vi "MasterAcquisitionFile_PCO_IOS_MultiWavelength.vi"() -> ()   [LabVIEW 2020]
uses:
  <userlib>/PCO LabVIEW 5.0.0/pco.camera/Controls/binning.ctl
  <vilib>/vision/driver/IMAQdx.llb/IMAQdx Acquisition Mode.ctl
  <vilib>/vision/driver/IMAQdx.llb/IMAQdx Camera Control Mode.ctl
  <vilib>/userDefined/High Color/IMAQdx.ctl
  <userlib>/PCO LabVIEW 5.0.0/pco.camera/Camera.lvclass
  <vilib>/vision/driver/IMAQdx.llb/IMAQdx Buffer Number Mode.ctl
  <vilib>/DAQmx/write.llb/DAQmx Write (Digital 1D Wfm NChan NSamp).vi
  <vilib>/DAQmx/write.llb/DAQmx Write (Digital Bool 1Line 1Point).vi
  <vilib>/DAQmx/read.llb/DAQmx Read (Analog 1D Wfm NChan NSamp).vi
  <vilib>/Waveform/DWDTOps.llb/DWDT Digital to Boolean Array.vi
  <vilib>/DAQmx/create/channels.llb/DAQmx Create Channel (CO-Pulse Generation-Frequency).vi
  <vilib>/DAQmx/configure/timing.llb/DAQmx Timing (Implicit).vi
  <vilib>/DAQmx/create/channels.llb/DAQmx Create Channel (AI-Voltage-Basic).vi
  <vilib>/DAQmx/configure/timing.llb/DAQmx Timing (Sample Clock).vi
  <vilib>/DAQmx/configure/trigger.llb/DAQmx Start Trigger (Digital Edge).vi
  <vilib>/DAQmx/create/channels.llb/DAQmx Create Channel (DO-Digital Output).vi
  <vilib>/Waveform/DWDTOps.llb/DWDT Boolean Array to Digital.vi
  <vilib>/Waveform/DWDTOps.llb/DWDT Uncompress Digital.vi
  <vilib>/DAQmx/miscellaneous.llb/DAQmx Fill In Error Info.vi
  <vilib>/vision/driver/NI_Vision_Acquisition_Software.lvlib
  <resource>/objmgr/imaqdx.rc
  <resource>/objmgr/daqmx.rc
panel:
  out "Recorded Images":u32
  in  "ROI":cluster{"x0":u64, "y0":u64, "x1":u64, "y1":u64}={"x0"=1, "y0"=1, "x1"=640, "y1"=540}
  in  "Binning":T1={"vert"=4, "horz"=4}
  in  "TriggerMode":T2(ring)=enum."external exposure start"
  in  "Exposure [s]":dbl=0.01 min=0.0005 max=2.0 step=0.001
  out "Image":T3(plugin-control)
  out "LED":bool
  out "Auditory":bool
  out "RPad":bool
  out "LPad":bool
  out "Finished":bool
  in  "Generate Stimuli":bool=TRUE
  in  "Sol Stim Parameters":cluster{"Fs":dbl, "Samples":dbl}
  in  "LED Stim Parameters":cluster{"Fs":dbl, "Samples":dbl}
  in  "Sol Duty Cycle (%)":dbl=50.0
  in  "Sol Freq":dbl=1.0
  in  "Sol Dur (s)":dbl=1.0
  in  "LED Duty Cycle (%)":dbl=10.0
  in  "LED Freq":dbl=10.0
  in  "LED Dur (s)":dbl=2.0
  out "Stimulus Order":digitalwaveform[](graph)=[{"t0"=timestamp(0 s since 1904-01-01), "dt"=5e-05, "Y"={"transitions"=[], "data"=array6001000x1[6001000 elements]}}, {"t0"=timestamp(0 s since 1904-01-01), "dt"=5e-05, "Y"={"transitions"=[], "data"=array6001000x1[6001000 elements]}}, {"t0"=timestamp(0 s since 1904-01-01), "dt"=5e-05, "Y"={"transitions"=[], "data"=array6001000x1[6001000 elements]}}, {"t0"=timestamp(0 s since 1904-01-01), "dt"=5e-05, "Y"={"transitions"=[], "data"=array6001000x1[6001000 elements]}}]
  out "Solenoid Stim":digitalwaveform(graph)={"t0"=timestamp(0 s since 1904-01-01), "dt"=5e-05, "Y"={"transitions"=[], "data"=array20000x1[20000 elements]}}
  in  "Trial Offset (s)":dbl=5.0
  in  "Interstim (s)":dbl=10.0
  in  "Right Pad":dbl=1.0
  in  "Left Pad":dbl=1.0
  in  "Auditory":dbl=1.0
  in  "LED":dbl
  out "?":T3(plugin-control)
  out "?":T3(plugin-control)
  out "?":T3(plugin-control)
  in  "stop":bool
  out "PCO":bool
  out "Pupil Cam":bool
  out "Whisk Cam":bool
  out "Web Cam":bool
  out "Analog":bool
  out "Web Cam Fs":dbl(knob) scale=0.0..200.0
  out "Whisk Cam Fs":dbl(knob) scale=0.0..200.0
  out "Last Whisk\nBuffer 2":u32=1
  out "Pupil Cam Fs":dbl(knob) scale=0.0..200.0
  out "Dropped 2":u32(slide) caption="Pupil Cam" scale=0.0..99.0
  out "Dev1 Samples":i32
  in  "Dev1 Analog Channels":string[](array[string])=["Cortical_LH", "Force_Sensor", "LPadSol", "RPadSol", "AudSol", "Hippocampus", "EMG", "Cortical_RH", "OptoLED"]
  in  "Analog Acquisition":cluster{"Analog Fs":u16}={"Analog Fs"=20000} {"Analog Fs" format="%0.0f"}
  in  "Sampling Rates":T4={"CBV Cam Fs"=30, "Whisk Cam Fs"=150, "Web Cam Fs"=30, "Pupil Cam Fs"=30}
  out "Notes Size":i32=8
  out "Notes Reversed":string[](array[string])=["Experimenter", "Animal ID", "Hemisphere", "Solenoid PSI", "Isoflurane time", "Session ID", "Amplifier Gain", "LED power (mW)"]
  out "Notes Array":string[](array[string])=["LED power (mW)", "Amplifier Gain", "Session ID", "Isoflurane time", "Solenoid PSI", "Hemisphere", "Animal ID", "Experimenter"]
  in  "Notes:":T5={"Experimenter"="Kevin", "Animal ID"="FS28", "Hemisphere"="LH", "Solenoid PSI"="10", "Isoflurane time"="1420", "Session ID"="Imaging Session One", "Amplifier Gain"="10000", "Opto LED (mW)"="10", "Wavelengths"="530 nm", "Lens mag"="1.5X"}
  in  "Target Path":path=path "D:/FS28/5 minute 530 only" caption="Final Save Location"
  out "Dropped":u32(slide) caption="Whisk Cam" scale=0.0..999.0
  out "Filename":string="230405_14_53_47"
  out "CBV Camera":bool=TRUE
  out "Time Elapsed (Min)":cluster{dbl, dbl}(slide)={15.0, 5.0010000000000004e-05} scale=0.0..15.0 scale format="%.1g"
  in  "Time (min)":dbl(knob)=15.0 min=0.5 max=20.0 step=0.5 scale=0.0..20.0 scale format="%#_2g"
  in  "Temp Path":path=path "D:/LabVIEW Streamed Data" caption="Temporary Path for Streamed Data"
  out "Last Whisk\nBuffer":u32=1
  # "PCO Parameters"
  # "Stimuli"
  # "LPAD"
  # "RPAD"
  # "AUD"
  # "LED"
  # "Dropped Frames"
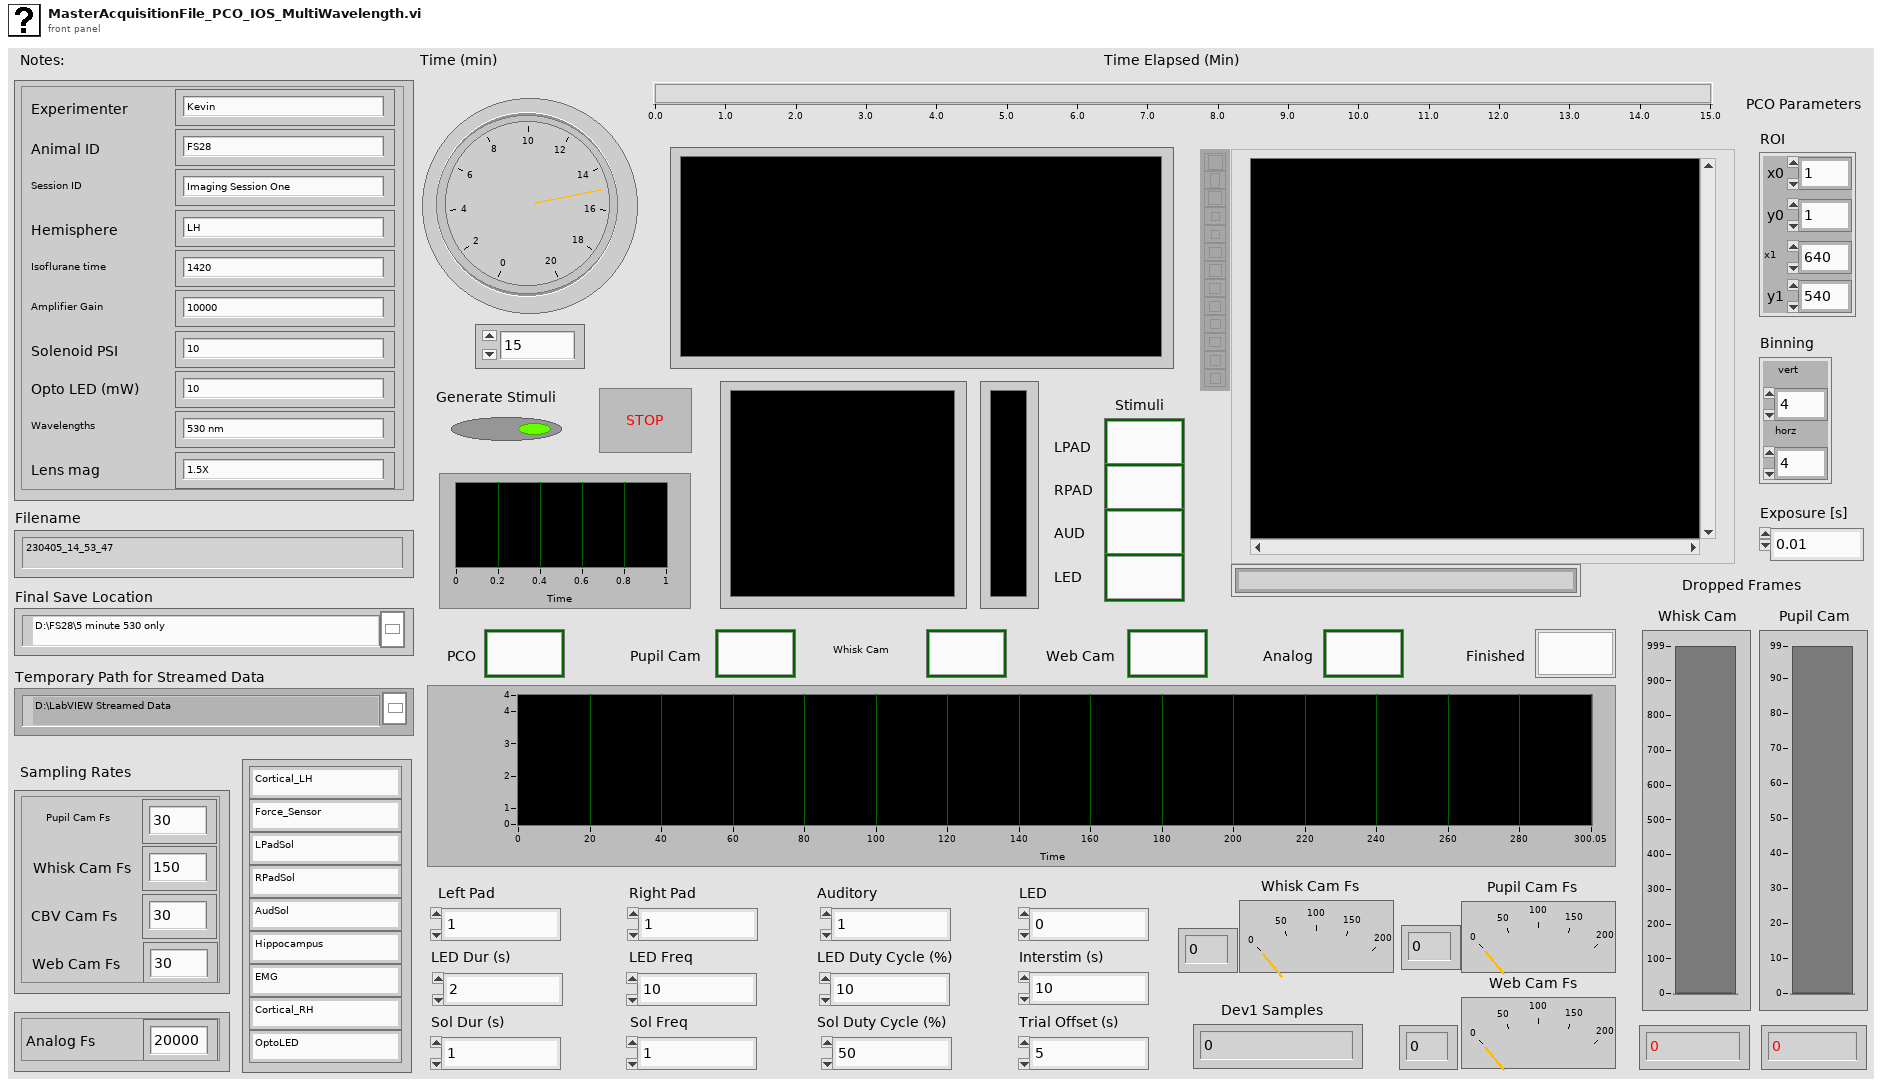
[diagram p1: front panel]
types:
  T1 = typedef "Camera.lvclass/binning.ctl" = cluster{"vert":u16, "horz":u16}
  T2 = enum16{"auto sequence", "software trigger", "external exposure start", "external exposure control"}
  T3 = typedef "IMAQ Image.ctl" = refnum<image>
  T4 = cluster{"CBV Cam Fs":u16, "Whisk Cam Fs":u16, "Web Cam Fs":u16, "Pupil Cam Fs":u16}
  T5 = cluster{"Experimenter":string, "Animal ID":string, "Hemisphere":string, "Solenoid PSI":string, "Isoflurane time":string, "Session ID":string, "Amplifier Gain":string, "Opto LED (mW)":string, "Wavelengths":string, "Lens mag":string}
  T6 = typedef "Image Type" = u32
  T7 = typedef "IMAQdx.ctl" = refnum<k21>
  T8 = enum16{"open", "replace", "create", "open or create", "replace or create", "replace or create with confirmation"}
  T9 = typedef "NI_Vision_Acquisition_Software.lvlib/IMAQdx Acquisition Mode.ctl" = enum32{"One Shot", "Continuous"}
  T10 = typedef "NI_Vision_Acquisition_Software.lvlib/IMAQdx Camera Control Mode.ctl" = enum32{"Controller", "Listener"}
  T11 = enum16{"open", "open or create", "create or replace", "create", "open (read-only)"}
  T12 = cluster{"exposure_time_s":dbl, "delay_time_s":dbl, "roi":cluster{"x0":u64, "y0":u64, "x1":u64, "y1":u64}, "timestamp_mode":u16, "pixelrate":u32, "trigger_mode":u16, "acquire_mode":u16, "metadata_mode":u16, "noisefilter_mode":u16, "binning":T1}
  T13 = typedef "IMAQ AVI2 Refnum.ctl" = refnum<k20>
  T14 = enum16{"sequence", "sequence non blocking", "ring buffer", "fifo", "sequence_dpcore", "sequence_non_blocking_dpcore", "ring_buffer_dpcore", "fifo_dpcore", "tif", "multitif", "pcoraw", "b16", "dicom", "multidicom"}
  T15 = enum16{"Undefined", "Mono8", "Mono16", "BGRA8", "RGBA8", "BGRA16", "RGBA16", "CompressedMono8"}
  T16 = enum16{"big-endian, network order", "native, host order", "little-endian"}
  T17 = typedef "NI_Vision_Acquisition_Software.lvlib/IMAQdx Buffer Number Mode.ctl" = enum32{"Next", "Last", "Buffer Number", "Every", "Last New"}
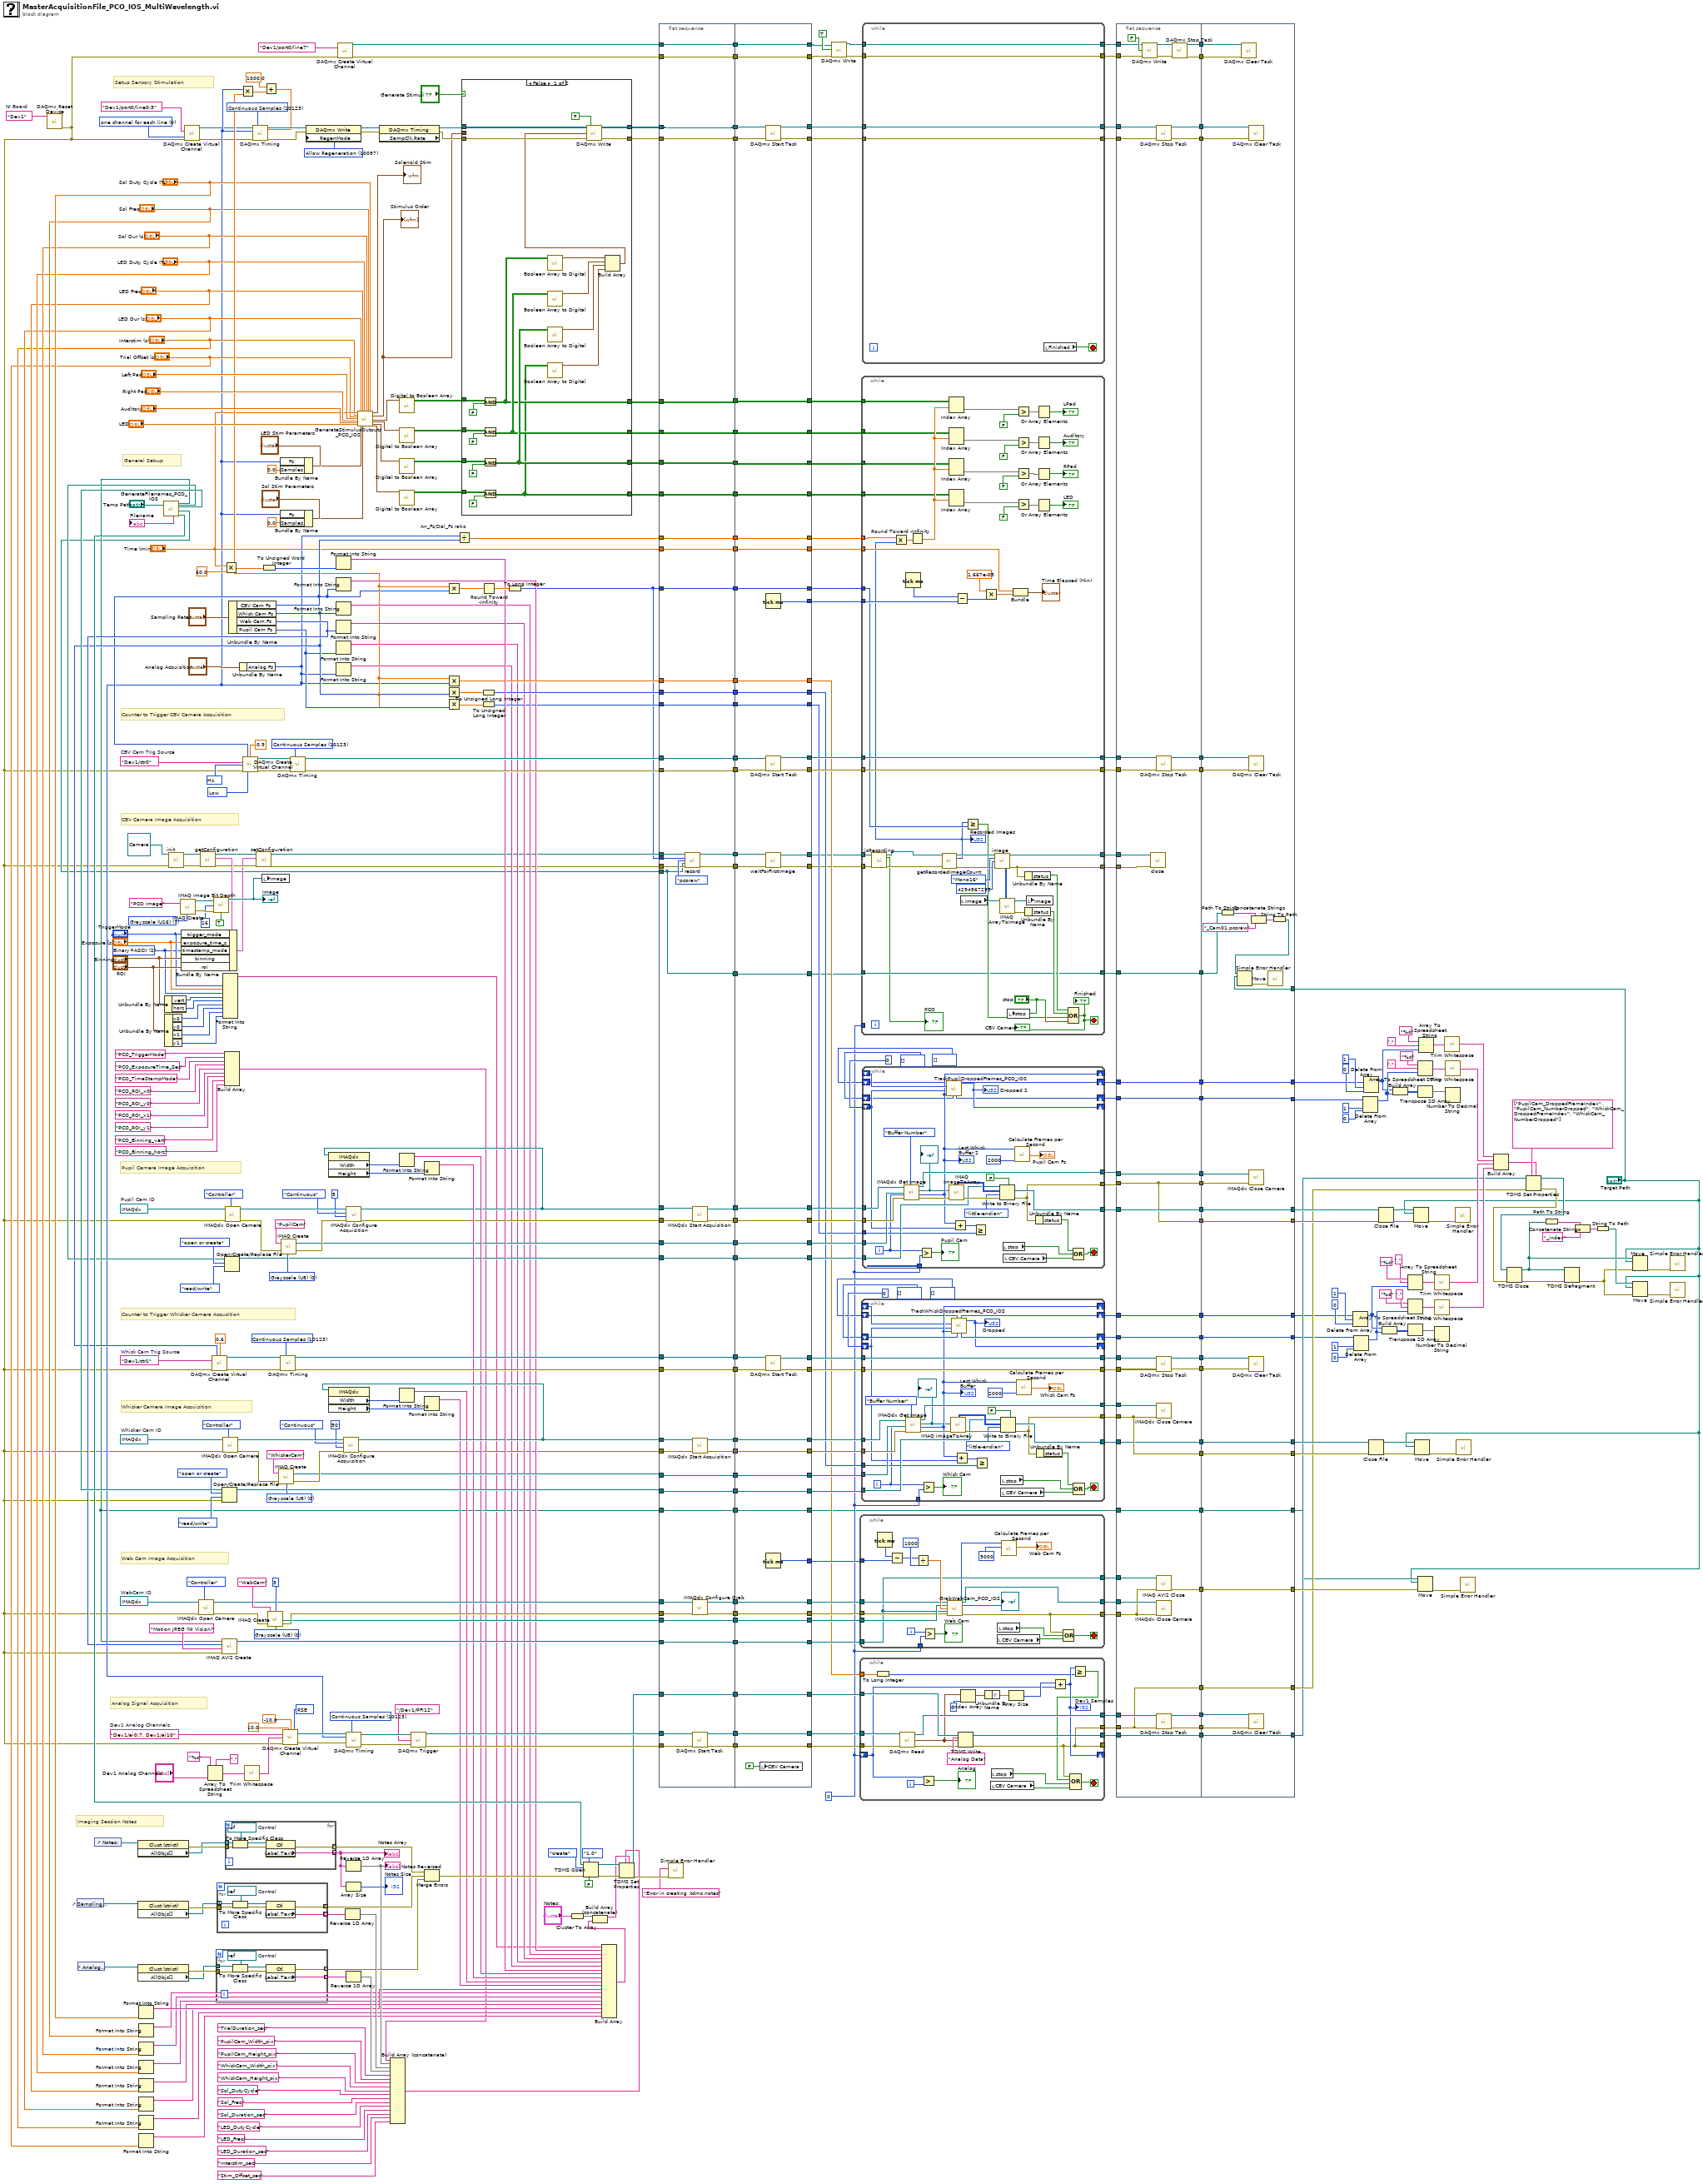
[diagram p0: block diagram]
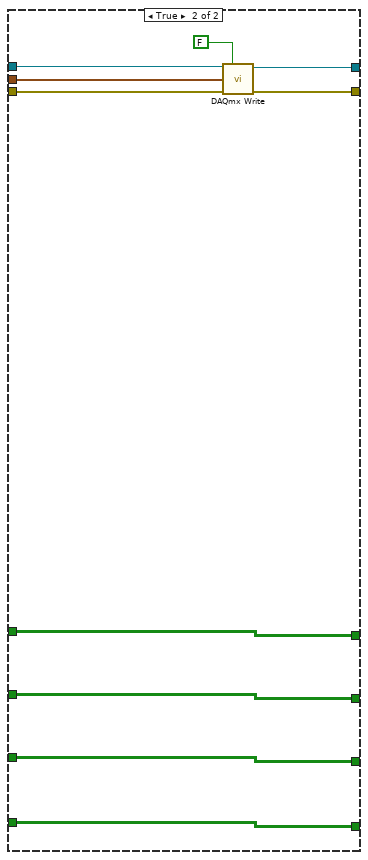
[diagram p2: hidden frame]
diagram:
  w39 = u16 2 items=["OFF", "Binary", "Binary+ASCII", "ASCII"] ("wTimeStampMode")
  w63 = T6 7 items=["Grayscale (U8)", "Grayscale (I16)", "Grayscale (SGL)", "Complex (CSG)", "RGB (U32)", "HSL (U32)", "RGB (U64)", "Grayscale (U16)"] ("Image Type")
  w155 = 10097 items=["Allow Regeneration"=10097, "Do Not Allow Regeneration"=10158] ("RegenMode")
  w156 = 10123 items=["Finite Samples"=10178, "Continuous Samples"=10123, "Hardware Timed Single Point"=12522] ("sample mode")
  w159 = 0 items=["one channel for each line", "one channel for all lines"] ("line grouping")
  w328 = tag "Dev1/ai0:7, Dev1/ai10"  # Dev1 Analog Channels
  w331 = T7 "cam3"  # WebCam ID
  w317 = T7 "cam1"  # Whisker Cam ID
  w455 = tag "Dev1/ctr1"  # Whisk Cam Trig Source
  w279 = T7 "cam2"  # Pupil Cam ID
  w121 = tag "Dev1/ctr0"  # CBV Cam Trig Source
  w282 = T6 0 items=["Grayscale (U8)", "Grayscale (I16)", "Grayscale (SGL)", "Complex (CSG)", "RGB (U32)", "HSL (U32)", "RGB (U64)", "Grayscale (U16)"] ("Image Type")
  w212 = 0
  w400 = 10123 items=["Finite Samples"=10178, "Continuous Samples"=10123, "Hardware Timed Single Point"=12522] ("sample mode")
  w403 = 10083 items=["default"=-1, "RSE"=10083, "NRSE"=10078, "Differential"=10106, "Pseudodifferential"=12529] ("input terminal configuration")
  w438 = T6 0 items=["Grayscale (U8)", "Grayscale (I16)", "Grayscale (SGL)", "Complex (CSG)", "RGB (U32)", "HSL (U32)", "RGB (U64)", "Grayscale (U16)"] ("Image Type")
  w445 = tag "Dev1"  # NI Board
  w446 = 10123 items=["Finite Samples"=10178, "Continuous Samples"=10123, "Hardware Timed Single Point"=12522] ("sample mode")
  w449 = 10373 items=["Hz"=10373] ("units")
  w450 = 10214 items=["High"=10192, "Low"=10214] ("idle state")
  w451 = 10123 items=["Finite Samples"=10178, "Continuous Samples"=10123, "Hardware Timed Single Point"=12522] ("sample mode")
  w458 = T6 0 items=["Grayscale (U8)", "Grayscale (I16)", "Grayscale (SGL)", "Complex (CSG)", "RGB (U32)", "HSL (U32)", "RGB (U64)", "Grayscale (U16)"] ("Image Type")
  # "General Set-up"
  # "Pupil Camera Image Acquisition"
  # "Whisker Camera Image Acquisition"
  # "Imaging Session Notes"
  # "Setup Sensory Stimulation"
  # "CBV Camera Image Acquisition"
  # "Counter to Trigger CBV Camera Acquisition"
  # "Counter to Trigger Whisker Camera Acqusition"
  # "Web Cam Image Acquisition"
  # "Analog Signal Acquisition"
  n1 = call <vilib>:"DAQmx Reset Device.vi"("device in"=w445) -> ("error out"=w14:errorcluster)  [unwired: 14 in]
  n2 = control-ref of="Sampling Rates"() -> (w337:refnum<vi>)
  n3 = control-ref of="Analog Acquisition"() -> (w336:refnum<vi>)
  n4 = control-ref of="Notes:"() -> (w358:refnum<vi>)
  n5 = property class="Clust (strict)"(reference=w358) -> (error out=w361:errorcluster, "AllObjs[]"=w295:refnum<vi>[])  [unwired: 1 in, 1 out]
  n6 = property class="Clust (strict)"(reference=w337) -> (error out=w356:errorcluster, "AllObjs[]"=w296:refnum<vi>[])  [unwired: 1 in, 1 out]
  n7 = property class="Clust (strict)"(reference=w336) -> (error out=w335:errorcluster, "AllObjs[]"=w294:refnum<vi>[])  [unwired: 1 in, 1 out]
  n8 = Format Into String("Sol Duty Cycle (%)") -> (resulting string=w189:string)  [unwired: 3 in, 1 out]
  n9 = Format Into String("Sol Freq") -> (resulting string=w188:string)  [unwired: 3 in, 1 out]
  n10 = Format Into String("Sol Dur (s)") -> (resulting string=w187:string)  [unwired: 3 in, 1 out]
  n11 = Format Into String("LED Duty Cycle (%)") -> (resulting string=w186:string)  [unwired: 3 in, 1 out]
  n12 = Format Into String("LED Freq") -> (resulting string=w185:string)  [unwired: 3 in, 1 out]
  n13 = Format Into String("LED Dur (s)") -> (resulting string=w184:string)  [unwired: 3 in, 1 out]
  n14 = Format Into String("Interstim (s)") -> (resulting string=w183:string)  [unwired: 3 in, 1 out]
  n15 = Format Into String("Trial Offset (s)") -> (resulting string=w182:string)  [unwired: 3 in, 1 out]
  n16 = call "GenerateFilenames_PCO_IOS.vi"("path"="Temp Path") -> ("TDMS Path"=w353:path, "PCO Path"=w20:path, "Basler Path"=w441:path, "WebCam Path"=w67:path, "Analog file name"=→"Filename":string, "Basler2 Path"=w278:path)  [unwired: 3 in, 2 out]
  n17 = Unbundle By Name("Binning") -> ("vert"=w38:u16, "horz"=w37:u16)
  n18 = Unbundle By Name("ROI") -> ("x0"=w36:u64, "y0"=w35:u64, "x1"=w34:u64, "y1"=w33:u64)
  n19 = call-dynamic "init.vi"("Camera in"=refnum<class "Camera.lvclass"> refnum ("PCOCamera in"), "error in (no error)"=w14) -> ("Camera out"=w56:refnum<class "Camera.lvclass">, "error out"=w55:errorcluster)  [unwired: 7 in]
  n20 = call "IMAQ Create"("Image Name"="PCO Image", "Image Type"=w63) -> ("New Image"=w62:T3, "error out"=w61:errorcluster)  [unwired: 3 in]
  n21 = call-poly <vilib>:"DAQmx Create Virtual Channel.vi"("lines"=tag "Dev1/port0/line0:3", "line grouping"=w159, "error in"=w14) -> ("task out"=w158:refnum<k21>, "error out"=w157:errorcluster)  [unwired: 11 in]
  n22 = call <vilib>:"IMAQdx Open Camera.vi"("Camera Control Mode"=IMAQdx_Camera_Control_Mode."Controller", "error in"=w14, "Session In"=w331) -> ("error out"=w434:errorcluster, "Session Out"=w432:T7)  [unwired: 7 in]
  n23 = call-dynamic "getConfiguration.vi"("error in (no error)"=w55, "Camera in"=w56) -> ("error out"=w54:errorcluster, "configuration"=w58:T12, "Camera out"=w57:refnum<class "Camera.lvclass">)  [unwired: 7 in]
  n24 = Bundle By Name(cluster=w58, "trigger_mode"="TriggerMode", "exposure_time_s"="Exposure [s]", "timestamp_mode"=w39, "binning"="Binning", "roi"="ROI") -> (w53:T12)
  n25 = Array To Spreadsheet String(delimiter (Tab)=",", array="Dev1 Analog Channels", 3:"%s" ("format string")) -> (spreadsheet string=w325:string)
  n26 = call "IMAQ Image Bit Depth"("Image"=w62, "Bit Depth (0)"=u32 16, "error in (no error)"=w61, "Get/Set Bit Depth? (Set)"=TRUE) -> ("Image Out"=w64:T3)  [unwired: 9 in, 2 out]
  "Image" <- w64
  n27 = for {
    tunnel: [w470] -> w333 mode=indexing
    tunnel: w335 -> [w469]
    tunnel: [w467] -> w334 mode=indexing
    tunnel: w294 -> [w466] mode=indexing
    w471 = refnum<vi> refnum  # Control
    n28 = To More Specific Class(target class=w471, reference=w466, error in=w469) -> (specific class reference=w472:refnum<vi>, error out=w468:errorcluster)
    n29 = property class="Ctl"(reference=w472, error in=w468) -> (error out=w467:errorcluster, "Label.Text"=w470:string)  [unwired: 1 out]
  }
  n30 = for {
    tunnel: [w477] -> w357 mode=indexing
    tunnel: w356 -> [w476]
    tunnel: [w474] -> w343 mode=indexing
    tunnel: w296 -> [w473] mode=indexing
    w478 = refnum<vi> refnum  # Control
    n31 = To More Specific Class(target class=w478, reference=w473, error in=w476) -> (specific class reference=w479:refnum<vi>, error out=w475:errorcluster)
    n32 = property class="Ctl"(reference=w479, error in=w475) -> (error out=w474:errorcluster, "Label.Text"=w477:string)  [unwired: 1 out]
  }
  n33 = Open/Create/Replace File(file path (use dialog)=w441, error in=w14, operation (0:open)=T8."open or create", access (0:read/write)=enum16{"read/write", "read-only", "write-only"}."read/write") -> (refnum out=w411:refnum<file>)  [unwired: 2 in, 2 out]
  n34 = Format Into String("TriggerMode", "Exposure [s]", w39, w38, w37, w36, w35, w34, w33) -> (resulting string=w31:string)  [unwired: 3 in, 1 out]
  n35 = call <vilib>:"IMAQdx Open Camera.vi"("Camera Control Mode"=IMAQdx_Camera_Control_Mode."Controller", "error in"=w14, "Session In"=w317) -> ("error out"=w461:errorcluster, "Session Out"=w464:T7)  [unwired: 7 in]
  n36 = Multiply(x="Time (min)", y=60.0) -> (x*y=w199:dbl)
  n37 = Build Array("PCO_TriggerMode", "PCO_ExposureTime_Sec", "PCO_TimeStampMode", "PCO_ROI_x0", "PCO_ROI_y0", "PCO_ROI_x1", "PCO_ROI_y1", "PCO_Binning_vert", "PCO_Binning_horz") -> (w32:string[])
  n38 = Open/Create/Replace File(file path (use dialog)=w278, operation (0:open)=T8."open or create", access (0:read/write)=enum16{"read/write", "read-only", "write-only"}."read/write") -> (refnum out=w263:refnum<file>)  [unwired: 3 in, 2 out]
  n39 = call <vilib>:"IMAQdx Open Camera.vi"("Camera Control Mode"=IMAQdx_Camera_Control_Mode."Controller", "error in"=w14, "Session In"=w279) -> ("error out"=w285:errorcluster, "Session Out"=w288:T7)  [unwired: 7 in]
  n40 = for {
    tunnel: [w484] -> w360 mode=indexing
    tunnel: w361 -> [w483]
    tunnel: [w481] -> w344 mode=indexing
    tunnel: w295 -> [w480] mode=indexing
    w485 = refnum<vi> refnum  # Control
    n41 = To More Specific Class(target class=w485, reference=w480, error in=w483) -> (specific class reference=w486:refnum<vi>, error out=w482:errorcluster)
    n42 = property class="Ctl"(reference=w486, error in=w482) -> (error out=w481:errorcluster, "Label.Text"=w484:string)  [unwired: 1 out]
  }
  "Notes Array" <- w360
  n43 = Unbundle By Name("Sampling Rates") -> ("CBV Cam Fs"=w200:u16, "Whisk Cam Fs"=w252:u16, "Web Cam Fs"=w330:u16, "Pupil Cam Fs"=w246:u16)
  n44 = call-poly <vilib>:"DAQmx Create Virtual Channel.vi"("frequency"=w252, "duty cycle"=0.6, "counter"=w455, "error in"=w14) -> ("task out"=w453:refnum<k21>, "error out"=w452:errorcluster)  [unwired: 10 in]
  n45 = call "IMAQ AVI2 Create"("error in (no error)"=w14, "Codec"="Motion JPEG (NI Vision)", "Frames Per Second"=w330, "AVI Path"=w67) -> ("AVI Refnum"=w424:T13)  [unwired: 6 in, 1 out]
  n46 = Unbundle By Name("Analog Acquisition") -> ("Analog Fs"=w172:u16)
  n47 = Multiply(x=w172, y=w199) -> (x*y=w132:dbl)
  n48 = call-poly <vilib>:"DAQmx Create Virtual Channel.vi"("frequency"=w200, "duty cycle"=0.9, "counter"=w121, "units"=w449, "error in"=w14, "idle state"=w450) -> ("task out"=w448:refnum<k21>, "error out"=w447:errorcluster)  [unwired: 8 in]
  n49 = call <vilib>:"Trim Whitespace.vi"("string"=w325) -> ("trimmed string"=w324:string)  [unwired: 1 in]
  n50 = call-dynamic "setConfiguration.vi"("error in (no error)"=w54, "configuration"=w53, "Camera in"=w57) -> ("error out"=w26:errorcluster, "Camera out"=w25:refnum<class "Camera.lvclass">)  [unwired: 7 in]
  n51 = To Unsigned Word Integer(number=w199) -> (unsigned 16bit integer=w320:u16)
  n52 = local write "Image"(w64) -> ()
  n53 = Add(x=1000.0, y=w132) -> (x+y=w130:dbl)
  n54 = call-poly <vilib>:"DAQmx Timing.vi"("task/channels in"=w158, "sample mode"=w156, "samples per channel"=w130, "rate"=w172, "error in"=w157) -> ("task out"=w152:refnum<k21>, "error out"=w151:errorcluster)  [unwired: 9 in]
  n55 = call "IMAQ Create"("Border Size"=3, "Image Name"="WebCam", "Image Type"=w438, "error in (no error)"=w434) -> ("New Image"=w431:T3, "error out"=w433:errorcluster)  [unwired: 1 in]
  n56 = call "IMAQ Create"("Image Name"="WhiskerCam", "Image Type"=w458, "error in (no error)"=w461) -> ("New Image"=w315:T3, "error out"=w459:errorcluster)  [unwired: 2 in]
  n57 = Bundle By Name(cluster="LED Stim Parameters", "Fs"=w172, "Samples"=0.0) -> (w205:cluster{"Fs":dbl, "Samples":dbl})
  n58 = Bundle By Name(cluster="Sol Stim Parameters", "Fs"=w172, "Samples"=0.0) -> (w206:cluster{"Fs":dbl, "Samples":dbl})
  n59 = call-poly <vilib>:"DAQmx Timing.vi"("task/channels in"=w453, "sample mode"=w451, "error in"=w452) -> ("task out"=w386:refnum<k21>, "error out"=w384:errorcluster)  [unwired: 11 in]
  n60 = call "IMAQ Create"("Image Name"="PupilCam", "Image Type"=w282, "error in (no error)"=w285) -> ("New Image"=w255:T3, "error out"=w283:errorcluster)  [unwired: 2 in]
  n61 = call-poly <vilib>:"DAQmx Create Virtual Channel.vi"("maximum value"=10.0, "minimum value"=-10.0, "input terminal configuration"=w403, "physical channels"=w328, "name to assign"=w324, "error in"=w14) -> ("task out"=w402:refnum<k21>, "error out"=w401:errorcluster)  [unwired: 8 in]
  n62 = call-poly <vilib>:"DAQmx Timing.vi"("task/channels in"=w448, "sample mode"=w446, "error in"=w447) -> ("task out"=w390:refnum<k21>, "error out"=w388:errorcluster)  [unwired: 11 in]
  n63 = property class="DAQmx Write"(reference=w152, error in=w151, "RegenMode"=w155) -> (reference out=w153:refnum<k21>, error out=w154:errorcluster)
  n64 = Format Into String(w320) -> (resulting string=w322:string)  [unwired: 3 in, 1 out]
  n65 = Format Into String(w200) -> (resulting string=w250:string)  [unwired: 3 in, 1 out]
  n66 = Format Into String(w252) -> (resulting string=w249:string)  [unwired: 3 in, 1 out]
  n67 = Format Into String(w330) -> (resulting string=w248:string)  [unwired: 3 in, 1 out]
  n68 = Format Into String(w246) -> (resulting string=w217:string)  [unwired: 3 in, 1 out]
  n69 = Format Into String(w172) -> (resulting string=w216:string)  [unwired: 3 in, 1 out]
  n70 = call-poly <vilib>:"DAQmx Create Virtual Channel.vi"("lines"=tag "Dev1/port0/line7", "error in"=w14) -> ("task out"=w12:refnum<k21>, "error out"=w10:errorcluster)  [unwired: 12 in]
  n71 = call <vilib>:"IMAQdx Configure Acquisition.vi"("error in"=w459, "Number of Buffers"=u32 50, "Continuous?"=IMAQdx_Acquisition_Mode."Continuous", "Session In"=w464) -> ("error out"=w224:errorcluster, "Session Out"=w316:T7)  [unwired: 6 in]
  n72 = property class="IMAQdx"(reference=w316) -> ("Width"=w319:u32, "Height"=w318:u32)  [unwired: 1 in, 2 out]
  n73 = Reverse 1D Array(array=w357) -> (reversed array=w347:string[])
  n74 = Reverse 1D Array(array=w360) -> (reversed array=w293:string[])
  "Notes Reversed" <- w293
  n75 = Array Size(array=w360) -> (size(s)=→"Notes Size":i32)
  n76 = Reverse 1D Array(array=w333) -> (reversed array=w332:string[])
  n77 = call <vilib>:"IMAQdx Configure Acquisition.vi"("error in"=w283, "Number of Buffers"=u32 5, "Continuous?"=IMAQdx_Acquisition_Mode."Continuous", "Session In"=w288) -> ("error out"=w265:errorcluster, "Session Out"=w256:T7)  [unwired: 6 in]
  n78 = property class="IMAQdx"(reference=w256) -> ("Width"=w277:u32, "Height"=w276:u32)  [unwired: 1 in, 2 out]
  n79 = call-poly <vilib>:"DAQmx Timing.vi"("task/channels in"=w402, "sample mode"=w400, "rate"=w172, "error in"=w401) -> ("task out"=w292:refnum<k21>, "error out"=w399:errorcluster)  [unwired: 10 in]
  n80 = call "GenerateStimulusOutputs_PCO_IOS.vi"("Trial duration (min)"="Time (min)", "Rest duration(s)"="Interstim (s)", "trial offset (s)"="Trial Offset (s)", "Left Pad"="Left Pad", "Right Pad"="Right Pad", "Auditory"="Auditory", "LED"="LED", "LED Stim Duration (s)"="LED Dur (s)", "LED Stim Parameters"=w205, "LED Frequency"="LED Freq", "Sol Stim Parameters"=w206, "LED duty cycle (%)"="LED Duty Cycle (%)", "Sol Stim Duration (s)"="Sol Dur (s)", "Sol Frequency"="Sol Freq", "Sol Duty Cycle (%)"="Sol Duty Cycle (%)") -> ("Solenoid Stim Waveforms"=→"Solenoid Stim":digitalwaveform, "Stimulus Digital Outputs"=w133:digitalwaveform[], "Left Pad Out"=w163:digitalwaveform, "Auditory Out"=w162:digitalwaveform, "Right Pad Out"=w161:digitalwaveform, "LED Out"=w160:digitalwaveform)  [unwired: 7 in]
  "Stimulus Order" <- w133
  n81 = property class="DAQmx Timing" props=["SampClk.Rate"](reference=w153, error in=w154) -> (reference out=w149:refnum<k21>, error out=w148:errorcluster)  [unwired: 1 out]
  n82 = Build Array (concatenate)(w32, w293, w347, w332, "TrialDuration_sec", "PupilCam_Width_pix", "PupilCam_Height_pix", "WhiskCam_Width_pix", "WhiskCam_Height_pix", "Sol_DutyCycle", "Sol_Freq", "Sol_Duration_sec", "LED_DutyCycle", "LED_Freq", "LED_Duration_sec", "Interstim_sec", "Stim_Offset_sec") -> (w290:string[])
  n83 = Format Into String(w277) -> (resulting string=w268:string)  [unwired: 3 in, 1 out]
  n84 = Format Into String(w319) -> (resulting string=w270:string)  [unwired: 3 in, 1 out]
  n85 = call-poly <vilib>:"Digital to Boolean Array.vi"("digital waveform"=w163) -> ("boolean array"=w141:bool[][])  [unwired: 9 in, 1 out]
  n86 = call-poly <vilib>:"Digital to Boolean Array.vi"("digital waveform"=w162) -> ("boolean array"=w140:bool[][])  [unwired: 9 in, 1 out]
  n87 = call-poly <vilib>:"Digital to Boolean Array.vi"("digital waveform"=w161) -> ("boolean array"=w139:bool[][])  [unwired: 9 in, 1 out]
  n88 = call-poly <vilib>:"Digital to Boolean Array.vi"("digital waveform"=w160) -> ("boolean array"=w138:bool[][])  [unwired: 9 in, 1 out]
  n89 = call-poly <vilib>:"DAQmx Trigger.vi"("task/channels in"=w292, "source"=tag "/Dev1/PFI12", "error in"=w399) -> ("task out"=w398:refnum<k21>, "error out"=w397:errorcluster)  [unwired: 11 in]
  n90 = Format Into String(w276) -> (resulting string=w269:string)  [unwired: 3 in, 1 out]
  n91 = Format Into String(w318) -> (resulting string=w271:string)  [unwired: 3 in, 1 out]
  n92 = Merge Errors(w344, w343, w334) -> (w342:errorcluster)
  n93 = Multiply(x=w199, y=w200) -> (x*y=w443:dbl)
  n94 = Multiply(x=w199, y=w172) -> (x*y=w306:dbl)
  n95 = Multiply(x=w252, y=w199) -> (x*y=w291:dbl)
  n96 = Multiply(x=w246, y=w199) -> (x*y=w251:dbl)
  n97 = Divide "An_Fs/Dal_Fs ratio"(x=w172, y=w200) -> (x/y=w116:dbl)
  n98 = case shown="False" "Generate Stimuli" {
    tunnel: w149 -> [w497 w518]
    tunnel: w148 -> [w496 w517]
    tunnel: [w494 w516] -> w146
    tunnel: [w495 w515] -> w144
    tunnel: w141 -> [w505 w514]
    tunnel: w140 -> [w506 w513]
    tunnel: w139 -> [w507 w512]
    tunnel: w138 -> [w508 w511]
    tunnel: [w489 w514] -> w137
    tunnel: [w490 w513] -> w136
    tunnel: [w491 w512] -> w135
    tunnel: [w487 w511] -> w134
    tunnel: w133 -> [_ w510]
    frame False {
      n99 = Compound Arithmetic op=AND(w505, FALSE) -> (w489:bool[][])
      n100 = Compound Arithmetic op=AND(w506, FALSE) -> (w490:bool[][])
      n101 = Compound Arithmetic op=AND(w507, FALSE) -> (w491:bool[][])
      n102 = Compound Arithmetic op=AND(w508, FALSE) -> (w487:bool[][])
      n103 = call-poly <vilib>:"Boolean Array to Digital.vi"("boolean array"=w489) -> ("digital waveform"=w499:digitalwaveform)  [unwired: 9 in, 1 out]
      n104 = call-poly <vilib>:"Boolean Array to Digital.vi"("boolean array"=w490) -> ("digital waveform"=w493:digitalwaveform)  [unwired: 9 in, 1 out]
      n105 = call-poly <vilib>:"Boolean Array to Digital.vi"("boolean array"=w491) -> ("digital waveform"=w492:digitalwaveform)  [unwired: 9 in, 1 out]
      n106 = call-poly <vilib>:"Boolean Array to Digital.vi"("boolean array"=w487) -> ("digital waveform"=w488:digitalwaveform)  [unwired: 9 in, 1 out]
      n107 = Build Array(w499, w493, w492, w488) -> (w498:digitalwaveform[])
      n108 = call-poly <vilib>:"DAQmx Write.vi"("task/channels in"=w497, "auto start"=FALSE, "data"=w498, "error in"=w496) -> ("task out"=w494:refnum<k21>, "error out"=w495:errorcluster)  [unwired: 9 in, 1 out]
    }
    frame True {
      n109 = call-poly <vilib>:"DAQmx Write.vi"("task/channels in"=w518, "auto start"=FALSE, "data"=w510, "error in"=w517) -> ("task out"=w516:refnum<k21>, "error out"=w515:errorcluster)  [unwired: 9 in, 1 out]
    }
  }
  n110 = To Unsigned Long Integer(number=w291) -> (unsigned 32bit integer=w304:u32)
  n111 = To Unsigned Long Integer(number=w251) -> (unsigned 32bit integer=w247:u32)
  n112 = Round Toward -Infinity(1:w443) -> (0:w442:dbl)
  n113 = To Long Integer(number=w442) -> (32bit integer=w24:i32)
  n114 = Cluster To Array(cluster="Notes:") -> (array=w354:string[])
  n115 = TDMS Open(6:FALSE ("disable buffering? (T)"), 7:enum16{"1.0", "2.0"}."1.0" ("file format version (2.0)"), 8:w342, 10:T11."create" ("operation (0:open)"), 11:w353) -> (0:w348:errorcluster, 3:w349:refnum<k34>)  [unwired: 2 in]
  n116 = Build Array(w31, w250, w249, w248, w217, w216, w322, w268, w269, w270, w271, w189, w188, w187, w186, w185, w184, w183, w182) -> (w329:string[])
  n117 = Build Array (concatenate)(w354, w329) -> (w346:string[])
  n118 = TDMS Set Properties(5:w346, 7:w290, 8:w348, 11:w349) -> (0:w341:errorcluster, 3:w345:refnum<k34>)  [unwired: 2 in, 2 out]
  n119 = flat-sequence {
    tunnel: w433 -> [w567]
    tunnel: w432 -> [w566]
    tunnel: w431 -> [w565]
    tunnel: [w565] -> w430
    tunnel: [w564] -> w428
    tunnel: [w563] -> w426
    tunnel: w424 -> [w562]
    tunnel: [w562] -> w423
    tunnel: w316 -> [w561]
    tunnel: w224 -> [w560]
    tunnel: [w559] -> w418
    tunnel: [w558] -> w416
    tunnel: [w557] -> w414
    tunnel: w315 -> [w557]
    tunnel: [w556] -> w412
    tunnel: w411 -> [w556]
    tunnel: w24 -> [w555]
    tunnel: [w555] -> w407
    tunnel: "Time (min)" -> [w554]
    tunnel: [w554] -> w404
    tunnel: w398 -> [w553]
    tunnel: w397 -> [w552]
    tunnel: [w551] -> w396
    tunnel: [w550] -> w395
    tunnel: [w549] -> w391
    tunnel: w345 -> [w549]
    tunnel: w390 -> [w548]
    tunnel: [w548] -> w389
    tunnel: w388 -> [w547]
    tunnel: [w547] -> w387
    tunnel: w386 -> [w546]
    tunnel: [w546] -> w385
    tunnel: w384 -> [w545]
    tunnel: [w545] -> w383
    tunnel: w306 -> [w544]
    tunnel: [w544] -> w305
    tunnel: w304 -> [w543]
    tunnel: [w543] -> w303
    tunnel: [w538] -> w267
    tunnel: w256 -> [w539]
    tunnel: [w536] -> w266
    tunnel: w265 -> [w537]
    tunnel: [w542] -> w264
    tunnel: w263 -> [w542]
    tunnel: w255 -> [w541]
    tunnel: [w541] -> w254
    tunnel: w247 -> [w540]
    tunnel: [w540] -> w245
    tunnel: [w535] -> w171
    tunnel: w137 -> [w535]
    tunnel: [w534] -> w170
    tunnel: w136 -> [w534]
    tunnel: [w533] -> w169
    tunnel: w135 -> [w533]
    tunnel: [w532] -> w168
    tunnel: w134 -> [w532]
    tunnel: [w531] -> w147
    tunnel: w146 -> [w531]
    tunnel: [w530] -> w145
    tunnel: w144 -> [w530]
    tunnel: w116 -> [w529]
    tunnel: [w529] -> w115
    tunnel: w67 -> [w528]
    tunnel: [w528] -> w68
    tunnel: [w527] -> w30
    tunnel: [w526] -> w29
    tunnel: w26 -> [w524]
    tunnel: w25 -> [w523]
    tunnel: w24 -> [w522]
    tunnel: w20 -> [w521]
    tunnel: [w521] -> w17
    tunnel: [w520] -> w13
    tunnel: w12 -> [w520]
    tunnel: [w519] -> w11
    tunnel: w10 -> [w519]
    tunnel: [w615] -> w435
    tunnel: w430 -> [w614]
    tunnel: [w614] -> w429
    tunnel: w428 -> [w613]
    tunnel: [w613] -> w427
    tunnel: w426 -> [w612]
    tunnel: [w612] -> w425
    tunnel: w423 -> [w611]
    tunnel: [w611] -> w422
    tunnel: [w596] -> w421
    tunnel: [w595] -> w420
    tunnel: [w610] -> w419
    tunnel: w418 -> [w610]
    tunnel: [w609] -> w417
    tunnel: w416 -> [w609]
    tunnel: [w608] -> w415
    tunnel: w414 -> [w608]
    tunnel: [w607] -> w413
    tunnel: w412 -> [w607]
    tunnel: [w600] -> w410
    tunnel: [w599] -> w409
    tunnel: [w606] -> w408
    tunnel: w407 -> [w605]
    tunnel: [w605] -> w406
    tunnel: [w604] -> w405
    tunnel: w404 -> [w604]
    tunnel: [w603] -> w393
    tunnel: w396 -> [w603]
    tunnel: [w602] -> w394
    tunnel: w395 -> [w602]
    tunnel: [w601] -> w214
    tunnel: w391 -> [w601]
    tunnel: w389 -> [w598]
    tunnel: w387 -> [w597]
    tunnel: w385 -> [w594]
    tunnel: w383 -> [w593]
    tunnel: w305 -> [w592]
    tunnel: [w592] -> w215
    tunnel: w303 -> [w591]
    tunnel: [w591] -> w244
    tunnel: w267 -> [w589]
    tunnel: w266 -> [w588]
    tunnel: w264 -> [w587]
    tunnel: [w589] -> w259
    tunnel: [w588] -> w258
    tunnel: [w587] -> w257
    tunnel: [w586] -> w253
    tunnel: w254 -> [w586]
    tunnel: [w585] -> w243
    tunnel: w245 -> [w585]
    tunnel: w171 -> [w581]
    tunnel: w170 -> [w584]
    tunnel: w169 -> [w583]
    tunnel: w168 -> [w582]
    tunnel: [w581] -> w167
    tunnel: [w584] -> w166
    tunnel: [w583] -> w165
    tunnel: [w582] -> w164
    tunnel: w147 -> [w580]
    tunnel: w145 -> [w579]
    tunnel: [w578] -> w143
    tunnel: [w577] -> w142
    tunnel: w115 -> [w576]
    tunnel: [w576] -> w114
    tunnel: [w575] -> w70
    tunnel: w68 -> [w575]
    tunnel: w30 -> [w574]
    tunnel: w29 -> [w573]
    tunnel: [w572] -> w28
    tunnel: [w571] -> w27
    tunnel: [w570] -> w16
    tunnel: w17 -> [w570]
    tunnel: w13 -> [w569]
    tunnel: w11 -> [w568]
    tunnel: [w569] -> w8
    tunnel: [w568] -> w7
    frame #0 {
      n120 = call-dynamic "record.vi"("Camera in"=w523, "num_images"=w522, "record_mode"=T14."pcoraw", "file_path"=w521, "error in (no error)"=w524) -> ("Camera out"=w527:refnum<class "Camera.lvclass">, "error out"=w526:errorcluster)  [unwired: 9 in]
      n121 = call <vilib>:"IMAQdx Start Acquisition.vi"("error in"=w537, "Session In"=w539) -> ("error out"=w536:errorcluster, "Session Out"=w538:T7)  [unwired: 8 in]
      n122 = call <vilib>:"IMAQdx Start Acquisition.vi"("error in"=w560, "Session In"=w561) -> ("error out"=w558:errorcluster, "Session Out"=w559:T7)  [unwired: 8 in]
      n123 = call <vilib>:"IMAQdx Configure Grab.vi"("error in"=w567, "Session In"=w566) -> ("error out"=w563:errorcluster, "Session Out"=w564:T7)  [unwired: 8 in]
      n124 = call <vilib>:"DAQmx Start Task.vi"("task/channels in"=w553, "error in"=w552) -> ("task out"=w551:refnum<k21>, "error out"=w550:errorcluster)  [unwired: 12 in]
    }
    frame #1 {
      n125 = local write "CBV Camera"(FALSE ("Finished Acquiring")) -> ()
      n126 = call-dynamic "waitForFirstImage.vi"("error in (no error)"=w573, "Camera in"=w574) -> ("error out"=w571:errorcluster, "Camera out"=w572:refnum<class "Camera.lvclass">)  [unwired: 8 in]
      n127 = call <vilib>:"DAQmx Start Task.vi"("task/channels in"=w580, "error in"=w579) -> ("task out"=w578:refnum<k21>, "error out"=w577:errorcluster)  [unwired: 12 in]
      n128 = Tick Count (ms)() -> (millisecond timer value=w606:u32)
      n129 = call <vilib>:"DAQmx Start Task.vi"("task/channels in"=w598, "error in"=w597) -> ("task out"=w600:refnum<k21>, "error out"=w599:errorcluster)  [unwired: 12 in]
      n130 = call <vilib>:"DAQmx Start Task.vi"("task/channels in"=w594, "error in"=w593) -> ("task out"=w596:refnum<k21>, "error out"=w595:errorcluster)  [unwired: 12 in]
      n131 = Tick Count (ms)() -> (millisecond timer value=w615:u32)
    }
  }
  n132 = call <vilib>:"Simple Error Handler.vi"("error source (\" \")"="Error in creating .tdms notes" ("error source (\" \")"), "error in (no error)"=w341) -> ()  [unwired: 3 in, 5 out]
  n133 = call-poly <vilib>:"DAQmx Write.vi"("task/channels in"=w8, "data"=TRUE, "error in"=w7) -> ("task out"=w4:refnum<k21>, "error out"=w2:errorcluster)  [unwired: 10 in, 1 out]
  n134 = while {
    tunnel: w394 -> [w638]
    tunnel: w393 -> [w637]
    tunnel: w214 -> [w636]
    tunnel: [w635] -> w85
    tunnel: [w624] -> _
    tunnel: [w634] -> w113
    shift-right: [w628] -> _
    shift-left: w212 -> [w619]
    tunnel: [w624] -> w112
    tunnel: w215 -> [w622]
    i -> [w620]
    stop <- w625 stop-if-true
    n135 = To Long Integer(number=w622) -> (32bit integer=w623:i32)
    n136 = call-poly <vilib>:"DAQmx Read.vi"("task/channels in"=w637, "error in"=w638) -> ("task out"=w634:refnum<k21>, "data"=w616:waveform(dbl)[], "error out"=w627:errorcluster)  [unwired: 11 in]
    n137 = Greater?(x=w619, y=w620) -> (0:→"Analog":bool)
    n138 = TDMS Write(0:w636, 5:"Analog Data" ("group name in (Untitled)"), 9:w616, 11:w627) -> (4:w635:refnum<k34>, 15:w624:errorcluster)  [unwired: 2 in, 2 out]
    n139 = Index Array(array=w616, index=0) -> (element=w631:waveform(dbl))
    n140 = Unbundle By Name(w631) -> ("Y"=w630:dbl[])
    n141 = local read "CBV Camera"() -> (w618:bool)
    n142 = local read "stop"() -> (w617:bool)
    n143 = Array Size(array=w630) -> (size(s)=w629:i32)
    n144 = Add(x=w629, y=w619) -> (x+y=w628:i32)
    "Dev1 Samples" <- w628
    n145 = Greater Or Equal?(x=w628, y=w623) -> (x >= y?=w626:bool)
    n146 = Compound Arithmetic op=OR(w624, w626, w617, w618) -> (w625:bool)
  }
  n147 = while {
    tunnel: w435 -> [w655]
    tunnel: w429 -> [w653]
    tunnel: w427 -> [w652]
    tunnel: w425 -> [w651]
    tunnel: w422 -> [w649]
    tunnel: [w650] -> w104
    tunnel: [w641] -> w105
    tunnel: [w649] -> w103
    tunnel: w212 -> [w644]
    i -> [w645]
    stop <- w642 stop-if-true
    n148 = Tick Count (ms)() -> (millisecond timer value=w657:u32)
    n149 = Subtract(x=w657, y=w655) -> (x-y=w658:u32)
    n150 = Divide(x=w658, y=u32 1000) -> (x/y=w654:dbl)
    n151 = Greater?(x=w645, y=w644) -> (0:→"Web Cam":bool)
    n152 = call "GrabWebCam_PCO_IOS.vi"("Session In"=w652, "Image In"=w653, "Trial Time"=w654, "AVI Refnum"=w649, "error in"=w651) -> ("Session Out"=w650:T7, "WebCam Img Out"=→"?":T3, "Buffer Number Out"=w648:u32, "error out"=w641:errorcluster)  [unwired: 7 in]
    n153 = local read "CBV Camera"() -> (w643:bool)
    n154 = local read "stop"() -> (w640:bool)
    n155 = call <vilib>:"Calculate Frames per Second.vi"("Update Interval (ms)"=u32 5000, "Buffer Number"=w648) -> ("Processed Frames/s"=→"Web Cam Fs":dbl)  [unwired: 7 in, 2 out]
    n156 = Compound Arithmetic op=OR(w641, w640, w643) -> (w642:bool)
  }
  n157 = while {
    tunnel: [w711] -> w125
    tunnel: w410 -> [w711]
    tunnel: [w710] -> w124
    tunnel: w409 -> [w710]
    tunnel: w408 -> [w709]
    tunnel: w406 -> [w665]
    tunnel: w405 -> [w708]
    tunnel: w212 -> [_]
    tunnel: w167 -> [w692]
    tunnel: w166 -> [w693]
    tunnel: w165 -> [w687]
    tunnel: w164 -> [w684]
    tunnel: w114 -> [w681]
    tunnel: w28 -> [w680]
    tunnel: w27 -> [w679]
    tunnel: [w669] -> w23
    tunnel: [w668] -> w22
    tunnel: [w661] -> w19
    tunnel: w16 -> [w661]
    stop <- w703 stop-if-true
    n158 = call-dynamic "isRecording.vi"("Camera in"=w680, "error in (no error)"=w679) -> ("Camera out"=w667:refnum<class "Camera.lvclass">, "recording"=→"PCO":bool, "error out"=w666:errorcluster)  [unwired: 11 in]
    n159 = Tick Count (ms)() -> (millisecond timer value=w714:u32)
    n160 = call-dynamic "getRecordedImageCount.vi"("Camera in"=w667, "error in (no error)"=w666) -> ("Camera out"=w673:refnum<class "Camera.lvclass">, "recorded_image_count"=w664:u32, "error out"=w672:errorcluster)  [unwired: 11 in]
    "Recorded Images" <- w664
    n161 = Multiply(x=w681, y=w664) -> (x*y=w704:dbl)
    n162 = Round Toward -Infinity(1:w704) -> (0:w698:dbl)
    n163 = Index Array(array=w692, index (row)=w698) -> (element=w691:bool[])  [unwired: 1 in]
    n164 = Index Array(array=w693, index (row)=w698) -> (element=w689:bool[])  [unwired: 1 in]
    n165 = Index Array(array=w687, index (row)=w698) -> (element=w686:bool[])  [unwired: 1 in]
    n166 = Index Array(array=w684, index (row)=w698) -> (element=w683:bool[])  [unwired: 1 in]
    n167 = Subtract(x=w714, y=w709) -> (x-y=w713:u32)
    n168 = local read "Image"() -> (w678:T3)
    n169 = Greater Or Equal?(x=w664, y=w665) -> (x >= y?=w670:bool)
    n170 = Multiply(x=w713, y=1.667e-05) -> (x*y=w712:dbl)
    n171 = call-dynamic "image.vi"("Camera in"=w673, "data_format"=T15."Mono16", "image_index"=u32 4294967295 ("dwImgIdx"), "error in (no error)"=w672) -> ("Camera out"=w669:refnum<class "Camera.lvclass">, "raw_image (U16)"=w677:u16[][], "error out"=w668:errorcluster)  [unwired: 4 in, 5 out]
    n172 = call "IMAQ ArrayToImage"("Image Pixels (U16)"=w677, "Image"=w678) -> ("error out"=w675:errorcluster, "Image Out"=w671:T3)  [unwired: 8 in]
    n173 = local write "stop"("stop") -> ()
    n174 = Bundle("Time (min)"=w708, w712) -> (→"Time Elapsed (Min)":cluster{"Time (min)":dbl, dbl})  [unwired: 1 in]
    n175 = Greater?(x=w691, y=FALSE ("Boolean")) -> (0:w690:bool[])
    n176 = Greater?(x=w689, y=FALSE ("Boolean")) -> (0:w688:bool[])
    n177 = Greater?(x=w686, y=FALSE ("Boolean")) -> (0:w685:bool[])
    n178 = Greater?(x=w683, y=FALSE ("Boolean")) -> (0:w682:bool[])
    n179 = Unbundle By Name(w668) -> ("status"=w662:bool)
    n180 = Unbundle By Name(w675) -> ("status"=w663:bool)
    n181 = local write "Image"(w671) -> ()
    n182 = Or Array Elements(Boolean array=w690) -> (logical OR=→"LPad":bool)
    n183 = Or Array Elements(Boolean array=w688) -> (logical OR=→"Auditory":bool)
    n184 = Or Array Elements(Boolean array=w685) -> (logical OR=→"RPad":bool)
    n185 = Or Array Elements(Boolean array=w682) -> (logical OR=→"LED":bool)
    n186 = Compound Arithmetic op=OR(w662, w663, w670, "stop") -> (w703:bool)
    "CBV Camera" <- w703
    "Finished" <- w703
  }
  n187 = while {
    tunnel: w421 -> [w741]
    tunnel: [w742] -> w108
    tunnel: w420 -> [w742]
    tunnel: [w741] -> w109
    tunnel: [w734] -> w99
    tunnel: [w735] -> w100
    tunnel: [w740] -> w95
    tunnel: w419 -> [w739]
    tunnel: w417 -> [w738]
    tunnel: w415 -> [w737]
    tunnel: w413 -> [w736]
    shift-right: [w725] -> _
    shift-left: _ -> [w723]
    shift-right: [w720] -> _
    shift-left: u32 0 ("New Lost") -> [w724]
    shift-right: [w721] -> w80
    shift-left: u32[] [] ("NewBuffNum") -> [w722]
    shift-right: [w727] -> w83
    shift-left: u32[] [] ("NewNumLost") -> [w726]
    tunnel: w244 -> [w732]
    tunnel: w212 -> [w728]
    i -> [w715]
    stop <- w731 stop-if-true
    n188 = call <vilib>:"IMAQdx Get Image.vi"("Buffer Number Mode (Next)"=IMAQdx_Buffer_Number_Mode."Buffer Number", "error in"=w738, "Buffer Number In"=w715, "Image In"=w737, "Session In"=w739) -> ("error out"=w748:errorcluster, "Buffer Number Out"=w725:u32, "Image Out"=w717:T3, "Session Out"=w734:T7)  [unwired: 3 in]
    "Last Whisk\nBuffer" <- w725
    "?" <- w717
    n189 = Greater?(x=w715, y=w728) -> (0:→"Whisk Cam":bool)
    n190 = call "IMAQ ImageToArray"("error in (no error)"=w748, "Image"=w717) -> ("error out"=w747:errorcluster, "Image Pixels (U8)"=w746:u8[][])  [unwired: 2 in, 3 out]
    n191 = call "TrackWhiskDroppedFrames_PCO_IOS.vi"("NumLost"=w726, "BuffNum"=w722, "Curr Buffer"=w725, "Prev Lost"=w724, "Prev Buffer"=w723) -> ("New Lost"=w720:u32, "NewNumLost"=w727:u32[], "NewBuffNum"=w721:u32[])  [unwired: 4 in]
    "Dropped" <- w720
    n192 = Add(x=w725, y=w724) -> (x+y=w733:u32)
    n193 = Greater Or Equal?(x=w733, y=w732) -> ()  [unwired: 1 out]
    n194 = Write to Binary File(file (use dialog)=w736, data=w746, error in=w747, 5:FALSE ("prepend array or string size? (T)"), 9:T16."little-endian" ("byte order (0:big-endian, network order)")) -> (refnum out=w740:refnum<file>, error out=w735:errorcluster)  [unwired: 1 in, 1 out]
    n195 = local read "stop"() -> (w719:bool)
    n196 = local read "CBV Camera"() -> (w718:bool)
    n197 = call <vilib>:"Calculate Frames per Second.vi"("Update Interval (ms)"=u32 2000, "Buffer Number"=w725) -> ("Processed Frames/s"=→"Whisk Cam Fs":dbl)  [unwired: 7 in, 2 out]
    n198 = Unbundle By Name(w735) -> ("status"=w716:bool)
    n199 = Compound Arithmetic op=OR(w716, w719, w718) -> (w731:bool)
  }
  n200 = while {
    tunnel: w143 -> [w752]
    tunnel: [w753] -> w128
    tunnel: w142 -> [w753]
    tunnel: [w752] -> w129
    tunnel: [w751] -> w3
    tunnel: w4 -> [w751]
    tunnel: w2 -> [w750]
    tunnel: [w750] -> w1
    stop <- w754 stop-if-true
    n201 = local read "Finished"() -> (w754:bool)
  }
  n202 = while {
    tunnel: [w769] -> w119
    tunnel: [w770] -> w118
    tunnel: [w779] -> w93
    tunnel: w259 -> [w778]
    tunnel: w258 -> [w777]
    tunnel: w253 -> [w776]
    tunnel: w257 -> [w775]
    shift-right: [w768] -> _
    shift-left: _ -> [w774]
    shift-right: [w773] -> _
    shift-left: u32 0 ("New Lost") -> [w767]
    shift-right: [w772] -> w74
    shift-left: u32[] [] ("NewBuffNum") -> [w763]
    shift-right: [w771] -> w77
    shift-left: u32[] [] ("NewNumLost") -> [w764]
    tunnel: w243 -> [w762]
    tunnel: w212 -> [w760]
    i -> [w755]
    stop <- w765 stop-if-true
    n203 = call <vilib>:"IMAQdx Get Image.vi"("Buffer Number Mode (Next)"=IMAQdx_Buffer_Number_Mode."Buffer Number", "error in"=w777, "Buffer Number In"=w755, "Image In"=w776, "Session In"=w778) -> ("error out"=w786:errorcluster, "Buffer Number Out"=w768:u32, "Image Out"=w757:T3, "Session Out"=w769:T7)  [unwired: 3 in]
    "Last Whisk\nBuffer 2" <- w768
    "?" <- w757
    n204 = Greater?(x=w755, y=w760) -> (0:→"Pupil Cam":bool)
    n205 = call "TrackPupilDroppedFrames_PCO_IOS.vi"("NumLost"=w764, "BuffNum"=w763, "Curr Buffer"=w768, "Prev Lost"=w767, "Prev Buffer"=w774) -> ("New Lost"=w773:u32, "NewNumLost"=w771:u32[], "NewBuffNum"=w772:u32[])  [unwired: 4 in]
    "Dropped 2" <- w773
    n206 = call "IMAQ ImageToArray"("error in (no error)"=w786, "Image"=w757) -> ("error out"=w785:errorcluster, "Image Pixels (U8)"=w784:u8[][])  [unwired: 2 in, 3 out]
    n207 = Add(x=w768, y=w767) -> (x+y=w766:u32)
    n208 = Greater Or Equal?(x=w766, y=w762) -> ()  [unwired: 1 out]
    n209 = Write to Binary File(file (use dialog)=w775, data=w784, error in=w785, 5:FALSE ("prepend array or string size? (T)"), 9:T16."little-endian" ("byte order (0:big-endian, network order)")) -> (refnum out=w779:refnum<file>, error out=w770:errorcluster)  [unwired: 1 in, 1 out]
    n210 = local read "stop"() -> (w759:bool)
    n211 = local read "CBV Camera"() -> (w758:bool)
    n212 = call <vilib>:"Calculate Frames per Second.vi"("Update Interval (ms)"=u32 2000, "Buffer Number"=w768) -> ("Processed Frames/s"=→"Pupil Cam Fs":dbl)  [unwired: 7 in, 2 out]
    n213 = Unbundle By Name(w770) -> ("status"=w756:bool)
    n214 = Compound Arithmetic op=OR(w756, w759, w758) -> (w765:bool)
  }
  n215 = flat-sequence {
    tunnel: w129 -> [w829]
    tunnel: w128 -> [w828]
    tunnel: [w827] -> w127
    tunnel: [w826] -> w126
    tunnel: w125 -> [w825]
    tunnel: w124 -> [w824]
    tunnel: [w823] -> w123
    tunnel: [w822] -> w122
    tunnel: [w821] -> w120
    tunnel: w119 -> [w821]
    tunnel: w118 -> [w805]
    tunnel: [w805] -> w117
    tunnel: w113 -> [w820]
    tunnel: w112 -> [w804]
    tunnel: [w819] -> w111
    tunnel: [w818] -> w110
    tunnel: w109 -> [w817]
    tunnel: w108 -> [w816]
    tunnel: [w815] -> _
    tunnel: [w814] -> _
    tunnel: [w815] -> w107
    tunnel: [w814] -> w106
    tunnel: w105 -> [w812]
    tunnel: w104 -> [w813]
    tunnel: w103 -> [w811]
    tunnel: [w810] -> w102
    tunnel: w100 -> [w808]
    tunnel: w99 -> [w809]
    tunnel: [w808] -> w97
    tunnel: [w807] -> w96
    tunnel: w95 -> [w807]
    tunnel: w93 -> [w806]
    tunnel: [w806] -> w92
    tunnel: [w805] -> w89
    tunnel: [w804] -> w88
    tunnel: w85 -> [w803]
    tunnel: [w803] -> w86
    tunnel: w83 -> [w802]
    tunnel: [w802] -> w82
    tunnel: w80 -> [w801]
    tunnel: [w801] -> w79
    tunnel: w77 -> [w800]
    tunnel: [w800] -> w76
    tunnel: w74 -> [w799]
    tunnel: [w799] -> w73
    tunnel: w70 -> [w798]
    tunnel: [w798] -> w69
    tunnel: w23 -> [w797]
    tunnel: w22 -> [w796]
    tunnel: w19 -> [w795]
    tunnel: [w795] -> w18
    tunnel: [w791] -> w6
    tunnel: [w790] -> w5
    tunnel: w3 -> [w789]
    tunnel: w1 -> [w788]
    tunnel: w127 -> [w860]
    tunnel: w126 -> [w859]
    tunnel: w123 -> [w858]
    tunnel: w122 -> [w857]
    tunnel: w120 -> [w856]
    tunnel: w117 -> [w855]
    tunnel: w111 -> [w854]
    tunnel: w110 -> [w853]
    tunnel: w107 -> [w852]
    tunnel: w106 -> [w851]
    tunnel: w102 -> [w850]
    tunnel: [w850] -> w101
    tunnel: [w849] -> w98
    tunnel: w97 -> [w849]
    tunnel: w96 -> [w848]
    tunnel: [w848] -> w94
    tunnel: w92 -> [w847]
    tunnel: [w847] -> w91
    tunnel: [w846] -> w90
    tunnel: w89 -> [w846]
    tunnel: w88 -> [w845]
    tunnel: [w845] -> w87
    tunnel: w86 -> [w844]
    tunnel: [w844] -> w84
    tunnel: w82 -> [w843]
    tunnel: [w843] -> w81
    tunnel: [w842] -> w78
    tunnel: w79 -> [w842]
    tunnel: w76 -> [w841]
    tunnel: [w841] -> w75
    tunnel: w73 -> [w840]
    tunnel: [w840] -> w72
    tunnel: [w839] -> w71
    tunnel: w69 -> [w839]
    tunnel: "Target Path" -> [w837]
    tunnel: w18 -> [w833]
    tunnel: w6 -> [w831]
    tunnel: w5 -> [w830]
    frame #0 {
      n216 = call-poly <vilib>:"DAQmx Write.vi"("task/channels in"=w789, "data"=FALSE, "error in"=w788) -> ("task out"=w793:refnum<k21>, "error out"=w794:errorcluster)  [unwired: 10 in, 1 out]
      n217 = call-dynamic "close.vi"("error in (no error)"=w796, "Camera in"=w797) -> ()  [unwired: 9 in, 1 out]
      n218 = call <vilib>:"DAQmx Stop Task.vi"("task/channels in"=w829, "error in"=w828) -> ("task out"=w827:refnum<k21>, "error out"=w826:errorcluster)  [unwired: 12 in]
      n219 = call <vilib>:"DAQmx Stop Task.vi"("task/channels in"=w825, "error in"=w824) -> ("task out"=w823:refnum<k21>, "error out"=w822:errorcluster)  [unwired: 12 in]
      n220 = call <vilib>:"DAQmx Stop Task.vi"("task/channels in"=w817, "error in"=w816) -> ("task out"=w815:refnum<k21>, "error out"=w814:errorcluster)  [unwired: 12 in]
      n221 = call <vilib>:"IMAQdx Close Camera.vi"("error in"=w808, "Session In"=w809) -> ()  [unwired: 9 in, 1 out]
      n222 = call "IMAQ AVI2 Close"("error in (no error)"=w812, "AVI Refnum"=w811) -> ("error out"=w810:errorcluster)  [unwired: 9 in]
      n223 = call <vilib>:"IMAQdx Close Camera.vi"("error in"=w812, "Session In"=w813) -> ()  [unwired: 9 in, 1 out]
      n224 = call <vilib>:"DAQmx Stop Task.vi"("task/channels in"=w820, "error in"=w804) -> ("task out"=w819:refnum<k21>, "error out"=w818:errorcluster)  [unwired: 12 in]
      n225 = call <vilib>:"DAQmx Stop Task.vi"("task/channels in"=w793, "error in"=w794) -> ("task out"=w790:refnum<k21>, "error out"=w791:errorcluster)  [unwired: 12 in]
    }
    frame #1 {
      n226 = Path To String(path=w833) -> (string=w836:string)
      n227 = call <vilib>:"DAQmx Clear Task.vi"("task in"=w830, "error in"=w831) -> ()  [unwired: 13 in, 1 out]
      n228 = call <vilib>:"DAQmx Clear Task.vi"("task in"=w860, "error in"=w859) -> ()  [unwired: 13 in, 1 out]
      n229 = call <vilib>:"DAQmx Clear Task.vi"("task in"=w858, "error in"=w857) -> ()  [unwired: 13 in, 1 out]
      n230 = call <vilib>:"IMAQdx Close Camera.vi"("error in"=w855, "Session In"=w856) -> ()  [unwired: 9 in, 1 out]
      n231 = call <vilib>:"DAQmx Clear Task.vi"("task in"=w852, "error in"=w851) -> ()  [unwired: 13 in, 1 out]
      n232 = call <vilib>:"DAQmx Clear Task.vi"("task in"=w854, "error in"=w853) -> ()  [unwired: 13 in, 1 out]
      n233 = Concatenate Strings(w836, "_Cam01.pcoraw" ("string")) -> (w834:string)
      n234 = String To Path(string=w834) -> (path=w832:path)
      n235 = Move(source path=w832, 10:w837) -> (error out=w838:errorcluster)  [unwired: 3 in, 2 out]
      n236 = call <vilib>:"Simple Error Handler.vi"("error in (no error)"=w838) -> ()  [unwired: 1 in, 8 out]
    }
  }
  n237 = Delete From Array(array=w78, length=1, index=0) -> (array with subset deleted=w298:u32[])  [unwired: 1 out]
  n238 = Delete From Array(array=w81, length=1, index=0) -> (array with subset deleted=w299:u32[])  [unwired: 1 out]
  n239 = Delete From Array(array=w75, length=1, index=0) -> (array with subset deleted=w230:u32[])  [unwired: 1 out]
  n240 = Delete From Array(array=w72, length=1, index=0) -> (array with subset deleted=w229:u32[])  [unwired: 1 out]
  n241 = Close File(refnum=w94, error in=w98) -> (path=w374:path, error out=w373:errorcluster)
  n242 = Close File(refnum=w91, error in=w90) -> (path=w226:path, error out=w225:errorcluster)
  n243 = Build Array(w298, w299) -> (w301:u32[][])
  n244 = Build Array(w229, w230) -> (w232:u32[][])
  n245 = Array To Spreadsheet String(delimiter (Tab)=",", array=w299, 3:"%d" ("format string")) -> (spreadsheet string=w307:string)
  n246 = Transpose 2D Array(2D array=w301) -> (transposed array=w300:u32[][])
  n247 = Array To Spreadsheet String(delimiter (Tab)=",", array=w298, 3:"%d" ("format string")) -> (spreadsheet string=w308:string)
  n248 = Move(source path=w226, error in=w225, 10:"Target Path") -> (error out=w227:errorcluster)  [unwired: 2 in, 2 out]
  n249 = Move(source path=w374, error in=w373, 10:"Target Path") -> (error out=w371:errorcluster)  [unwired: 2 in, 2 out]
  n250 = Array To Spreadsheet String(delimiter (Tab)=",", array=w230, 3:"%d" ("format string")) -> (spreadsheet string=w233:string)
  n251 = Transpose 2D Array(2D array=w232) -> (transposed array=w231:u32[][])
  n252 = Move(source path=w71, error in=w101, 10:"Target Path") -> (error out=w370:errorcluster)  [unwired: 2 in, 2 out]
  n253 = Array To Spreadsheet String(delimiter (Tab)=",", array=w229, 3:"%d" ("format string")) -> (spreadsheet string=w234:string)
  n254 = call <vilib>:"Trim Whitespace.vi"("string"=w308) -> ("trimmed string"=w220:string)  [unwired: 1 in]
  n255 = call <vilib>:"Trim Whitespace.vi"("string"=w307) -> ("trimmed string"=w219:string)  [unwired: 1 in]
  n256 = Number To Decimal String(number=w300) -> ()  [unwired: 1 in, 1 out]
  n257 = call <vilib>:"Trim Whitespace.vi"("string"=w234) -> ("trimmed string"=w221:string)  [unwired: 1 in]
  n258 = call <vilib>:"Trim Whitespace.vi"("string"=w233) -> ("trimmed string"=w222:string)  [unwired: 1 in]
  n259 = Number To Decimal String(number=w231) -> ()  [unwired: 1 in, 1 out]
  n260 = call <vilib>:"Simple Error Handler.vi"("error in (no error)"=w227) -> ()  [unwired: 1 in, 8 out]
  n261 = call <vilib>:"Simple Error Handler.vi"("error in (no error)"=w371) -> ()  [unwired: 1 in, 8 out]
  n262 = call <vilib>:"Simple Error Handler.vi"("error in (no error)"=w370) -> ()  [unwired: 1 in, 8 out]
  n263 = Build Array(w221, w222, w220, w219) -> (w218:string[])
  n264 = TDMS Set Properties(5:w218, 7:string[] ["PupilCam_DroppedFrameIndex", "PupilCam_NumberDropped", "WhiskCam_DroppedFrameIndex", "WhiskCam_NumberDropped"] ("channel name(s) in (Untitled)"), 8:w87, 11:w84) -> (0:w314:errorcluster, 3:w313:refnum<k34>)  [unwired: 2 in, 2 out]
  n265 = TDMS Close(8:w314, 11:w313) -> (0:w375:errorcluster, 3:w367:path)
  n266 = Path To String(path=w367) -> (string=w369:string)
  n267 = TDMS Defragment(4:w375, 7:w367) -> (0:w364:errorcluster)
  n268 = Concatenate Strings(w369, "_index" ("string")) -> (w366:string)
  n269 = String To Path(string=w366) -> (path=w365:path)
  n270 = Move(source path=w367, error in=w364, 10:"Target Path") -> (error out=w372:errorcluster)  [unwired: 2 in, 2 out]
  n271 = Move(source path=w365, error in=w364, 10:"Target Path") -> (error out=w228:errorcluster)  [unwired: 2 in, 2 out]
  n272 = call <vilib>:"Simple Error Handler.vi"("error in (no error)"=w372) -> ()  [unwired: 1 in, 8 out]
  n273 = call <vilib>:"Simple Error Handler.vi"("error in (no error)"=w228) -> ()  [unwired: 1 in, 8 out]
